vi "Problem 22.vi"() -> ()   [LabVIEW 2013, in "Problem 22.lvlib"]
uses:
  Problem 22.lvlib
  <vilib>/Utility/file.llb/Read From Spreadsheet File (string).vi
panel:
  out "Sum of Scores":i32
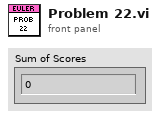
[diagram p1: front panel]
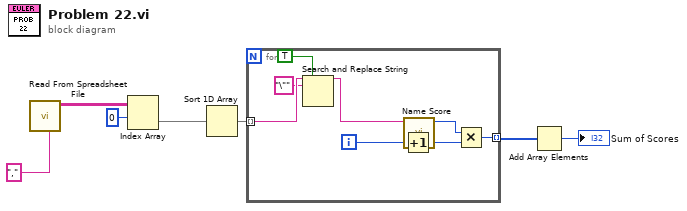
[diagram p0: block diagram]
diagram:
  n1 = call-poly <vilib>:"Read From Spreadsheet File.vi"("delimiter (\\t)"="," ("delimiter (\\t)")) -> ("all rows"=w6:string[][])  [unwired: 6 in, 4 out]
  n2 = Index Array(array=w6, index (row)=0) -> (element=w4:string[])  [unwired: 1 in]
  n3 = Sort 1D Array(array=w4) -> (sorted array=w3:string[])
  n4 = for {
    tunnel: w3 -> [w11] mode=indexing
    tunnel: [w12] -> w2 mode=indexing
    i -> [w14]
    n5 = Search and Replace String(replace all?=TRUE ("replace all? (F)"), input string=w11, search string="\"") -> (result string=w8:string)  [unwired: 5 in, 3 out]
    n6 = Increment(x=w14) -> (x+1=w13:i32)
    n7 = call "Name Score.vi"("Name"=w8) -> ("Name Score"=w15:i32)  [unwired: 10 in]
    n8 = Multiply(x=w15, y=w13) -> (x*y=w12:i32)
  }
  n9 = Add Array Elements(numeric array=w2) -> (sum=→"Sum of Scores":i32)
